vi "4461 - Create IO Channels Parallel Uneven.vi"(8 "error in":errorcluster, 11 "LockinDAQ":refnum<class "LockinDAQ.lvclass">) -> (0 "error out":errorcluster, 3 "LockinDAQ out":refnum<class "LockinDAQ.lvclass">)   [LabVIEW 2016, in "LockinDAQ.lvclass"]
uses:
  LockinDAQ.lvclass
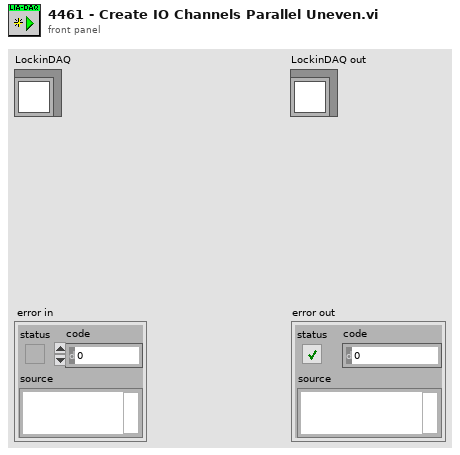
[diagram p1: front panel]
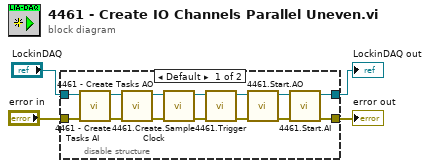
[diagram p0: block diagram]
diagram:
  n1 = disable-structure shown="Default" {
    disable-tunnel: "LockinDAQ" -> [w8 w20]
    disable-tunnel: "error in" -> [w7 w19]
    disable-tunnel: [w6 w20] -> w2
    disable-tunnel: [w5 w19] -> w1
    frame condition #0 (active) {
      n2 = call "4461 - Create Tasks AI.vi"("error in (no error)"=w7, "LockinDAQ"=w8) -> ("error out"=w9:errorcluster, "LockinDAQ out"=w10:refnum<class "LockinDAQ.lvclass">)  [unwired: 8 in]
      n3 = call "4461 - Create Tasks AO.vi"("error in (no error)"=w9, "LockinDAQ"=w10) -> ("error out"=w11:errorcluster, "LockinDAQ out"=w12:refnum<class "LockinDAQ.lvclass">)  [unwired: 8 in]
      n4 = call "4461.Create.Sample Clock.vi"("error in (no error)"=w11, "LockinDAQ"=w12) -> ("error out"=w13:errorcluster, "LockinDAQ out"=w14:refnum<class "LockinDAQ.lvclass">)  [unwired: 8 in]
      n5 = call "4461.Trigger.vi"("error in (no error)"=w13, "LockinDAQ"=w14) -> ("error out"=w18:errorcluster, "LockinDAQ out"=w15:refnum<class "LockinDAQ.lvclass">)  [unwired: 8 in]
      n6 = call "4461.Start.AO.vi"("error in (no error)"=w18, "LockinDAQ"=w15) -> ("error out"=w17:errorcluster, "LockinDAQ out"=w16:refnum<class "LockinDAQ.lvclass">)  [unwired: 8 in]
      n7 = call "4461.Start.AI.vi"("error in (no error)"=w17, "LockinDAQ"=w16) -> ("error out"=w5:errorcluster, "LockinDAQ out"=w6:refnum<class "LockinDAQ.lvclass">)  [unwired: 6 in]
    }
    frame condition #1 {
    }
  }
  "error out" <- w1
  "LockinDAQ out" <- w2
